vi "exnSharedSub floating point functions.vi"() -> (8 "yield floating point results":string[](array[string])=["acos(", "acosh(", "asin(", "asinh(", "atan(", "atanh(", "ci(", "cosh(", "cot(", "csc(", "expm1(", "gamma(", "getexp(", "getman(", "lnp1(", "rand(", "sec(", "si(", "sinc(", "sinh(", "spike(", "step(", "tanh(", "pi", "sqrt(", "log(", "log2(", "exp(", "ln(", "sin(", "cos(", "tan("])   [LabVIEW 2017]
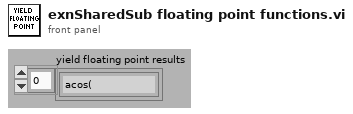
[diagram p1: front panel]
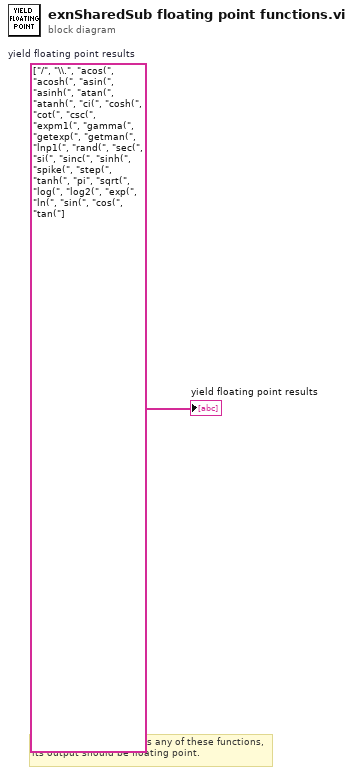
[diagram p0: block diagram]
diagram:
  w1 = string[] ["/", "\\.", "acos(", "acosh(", "asin(", "asinh(", "atan(", "atanh(", "ci(", "cosh(", "cot(", "csc(", "expm1(", "gamma(", "getexp(", "getman(", "lnp1(", "rand(", "sec(", "si(", "sinc(", "sinh(", "spike(", "step(", "tanh(", "pi", "sqrt(", "log(", "log2(", "exp(", "ln(", "sin(", "cos(", "tan("]  # yield floating point results
  # "If the Formula Node uses any of these functions, its output should be floating point."
  "yield floating point results" <- w1
